vi "LED State Implem.vi"(1 "LED State":T1(ring)=enum."Balancing") -> ()   [LabVIEW 2020]
uses:
  <vilib>/Rock Robotics/WPI/DriverStation/WPI_DriverStationRobotMode2.ctl
  <vilib>/Rock Robotics/Network Tables/NT Read Boolean.vi
  <vilib>/Rock Robotics/Network Tables/NT Read Number.vi
  Robot Global Data.vi
panel:
  out "size(s)":i32
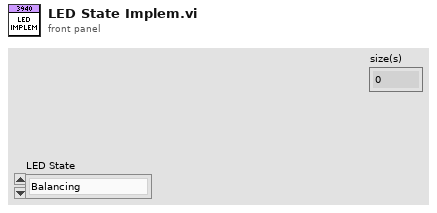
[diagram p1: front panel]
types:
  T1 = enum16{"Default", "Cone", "Cube", "Acquired", "Auto Red", "Auto Blue", "Balancing"}
  T2 = typedef "WPI_DriverStationRobotMode2.ctl" = enum16{"Autonomous Disabled", "Autonomous Enabled", "Teleop Disabled", "Teleop Enabled", "Disconnected", "Finish", "Test Disabled", "Test Enabled", "Emergency Stopped"}
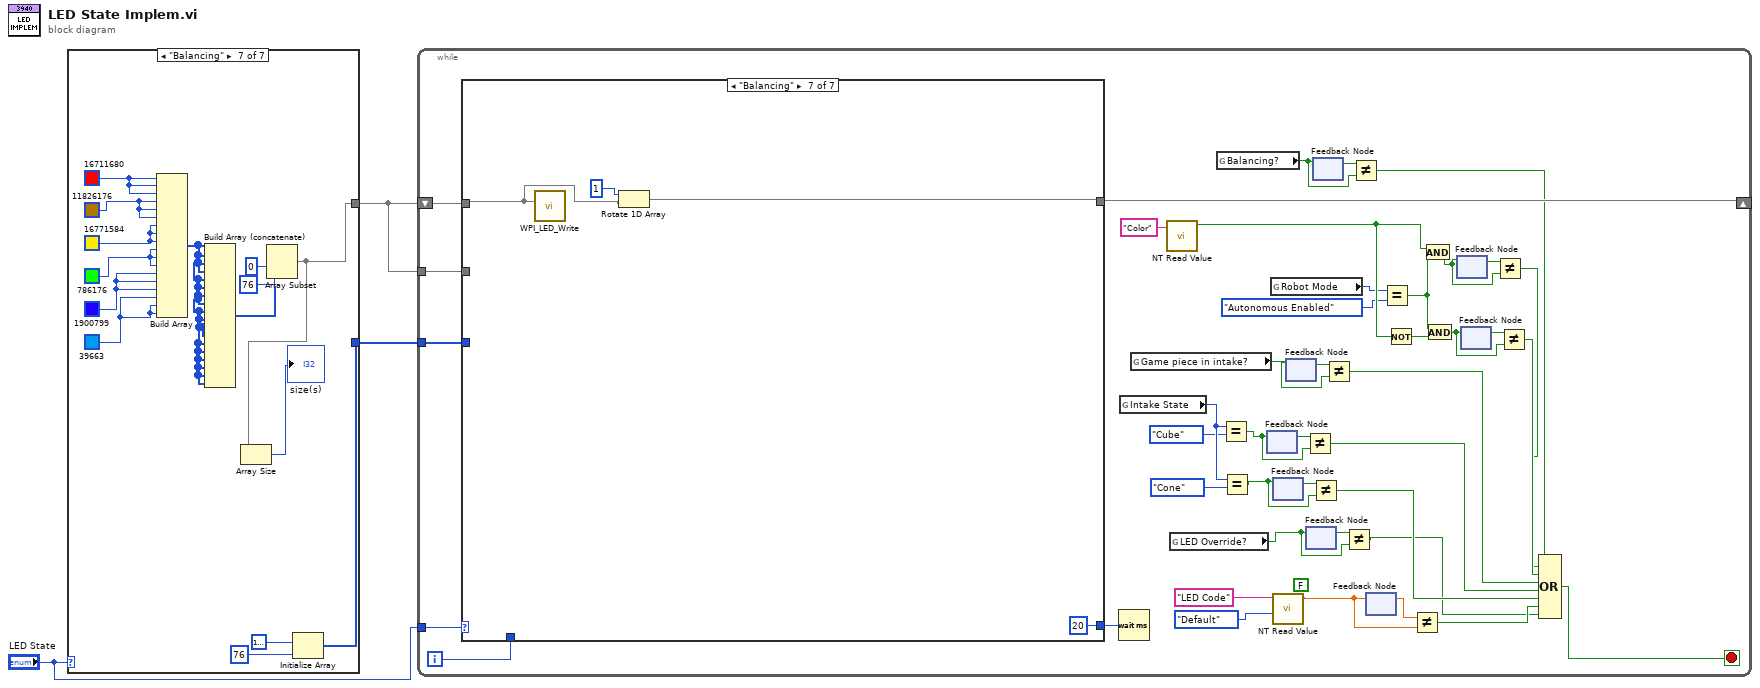
[diagram p0: block diagram]
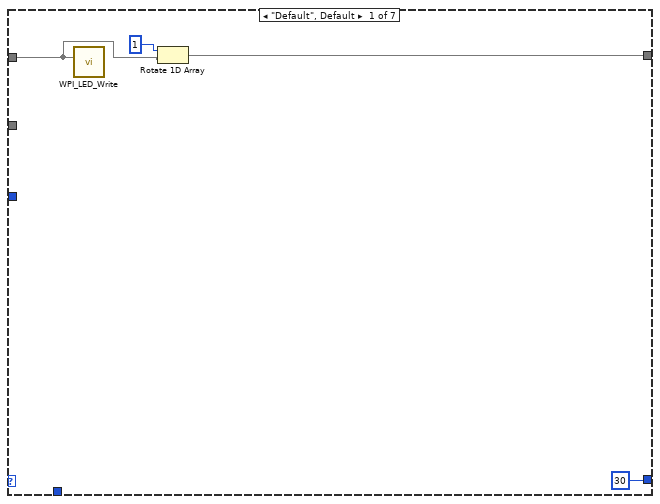
[diagram p2: hidden frame]
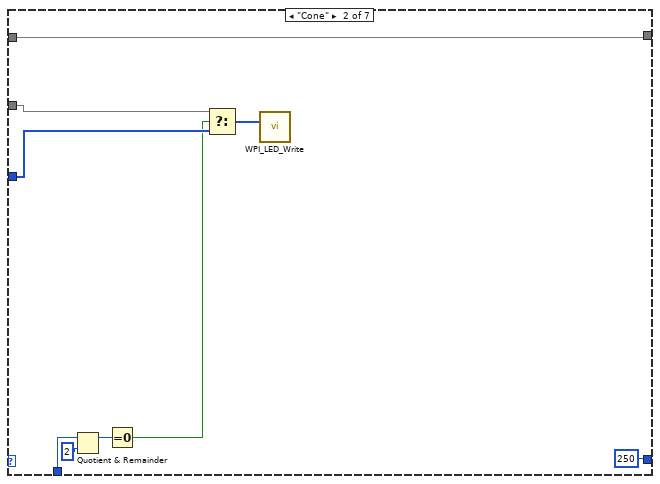
[diagram p3: hidden frame]
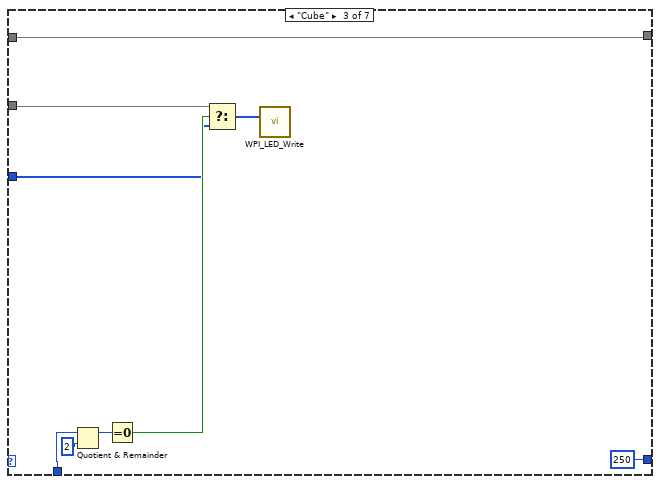
[diagram p4: hidden frame]
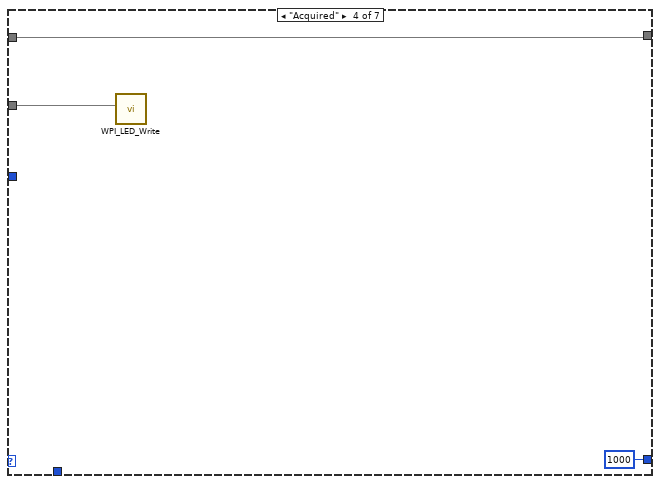
[diagram p5: hidden frame]
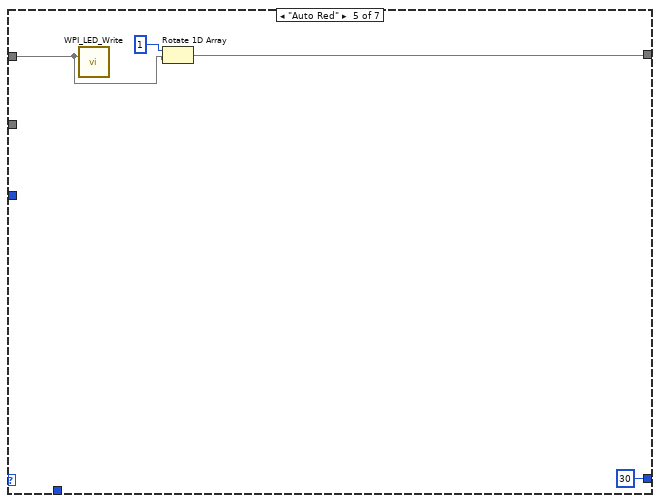
[diagram p6: hidden frame]
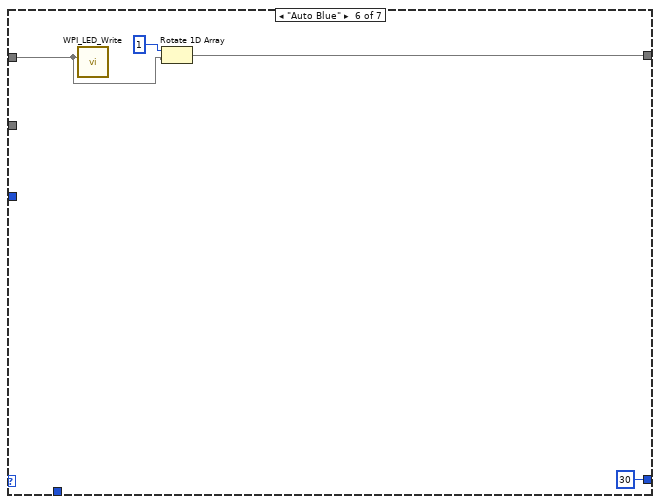
[diagram p7: hidden frame]
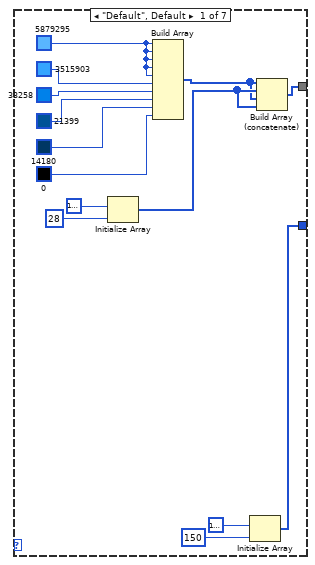
[diagram p8: hidden frame]
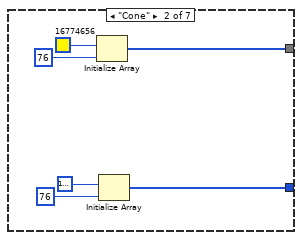
[diagram p9: hidden frame]
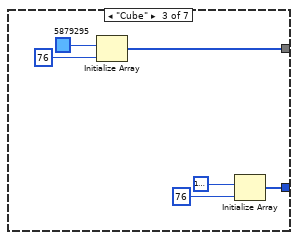
[diagram p10: hidden frame]
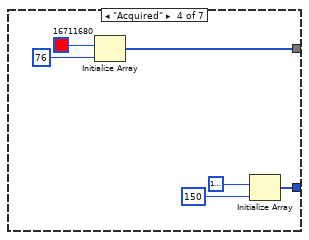
[diagram p11: hidden frame]
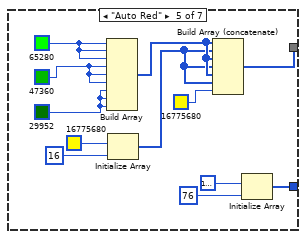
[diagram p12: hidden frame]
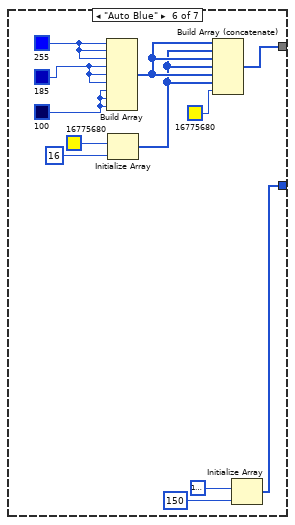
[diagram p13: hidden frame]
diagram:
  n1 = case shown="\"Balancing\"" "LED State" {
    tunnel: [w15 w21 w27 w33 w39 w51 w60] -> w2
    tunnel: [w12 w18 w24 w30 w45 w57 w72] -> w1
    frame "Default", Default {
      w11 = u32 5879295
      n2 = Initialize Array(u32 16777216, 28 ("dimension size")) -> (w5:u32[])
      n3 = Build Array(w11, w11, w11, w11, w11, u32 3515903, u32 33258, u32 21399, u32 14180, u32 0) -> (w4:u32[])
      n4 = Initialize Array(u32 16777216, 150 ("dimension size")) -> (w12:u32[])
      n5 = Build Array (concatenate)(w4, w5, w4, w5) -> (w15:u32[])
    }
    frame "Cone" {
      n6 = Initialize Array(u32 16774656, 76 ("dimension size")) -> (w21:u32[])
      n7 = Initialize Array(u32 16777216, 76 ("dimension size")) -> (w18:u32[])
    }
    frame "Cube" {
      n8 = Initialize Array(u32 5879295, 76 ("dimension size")) -> (w27:u32[])
      n9 = Initialize Array(u32 16777216, 76 ("dimension size")) -> (w24:u32[])
    }
    frame "Acquired" {
      n10 = Initialize Array(u32 16711680, 76 ("dimension size")) -> (w33:u32[])
      n11 = Initialize Array(u32 16777216, 150 ("dimension size")) -> (w30:u32[])
    }
    frame "Auto Red" {
      w42 = u32 29952
      w43 = u32 47360
      w44 = u32 65280
      n12 = Build Array(w44, w44, w44, w43, w43, w43, w42, w42, w42) -> (w38:u32[])
      n13 = Initialize Array(u32 16775680, 16 ("dimension size")) -> (w37:u32[])
      n14 = Build Array (concatenate)(w38, w37, w38, w37, w38, w37, u32 16775680) -> (w39:u32[])
      n15 = Initialize Array(u32 16777216, 76 ("dimension size")) -> (w45:u32[])
    }
    frame "Auto Blue" {
      w54 = u32 100
      w55 = u32 185
      w56 = u32 255
      n16 = Build Array(w56, w56, w56, w55, w55, w55, w54, w54, w54) -> (w50:u32[])
      n17 = Initialize Array(u32 16775680, 16 ("dimension size")) -> (w49:u32[])
      n18 = Build Array (concatenate)(w50, w49, w50, w49, w50, w49, u32 16775680) -> (w51:u32[])
      n19 = Initialize Array(u32 16777216, 150 ("dimension size")) -> (w57:u32[])
    }
    frame "Balancing" {
      w66 = u32 39663
      w67 = u32 1900799
      w68 = u32 786176
      w69 = u32 16771584
      w70 = u32 11826176
      w71 = u32 16711680
      n20 = Build Array(w71, w71, w71, w70, w70, w70, w69, w69, w69, w68, w68, w68, w67, w67, w67, w66, w66, w66) -> (w61:u32[])
      n21 = Build Array (concatenate)(w61, w61, w61, w61, w61, w61, w61, w61, w61, w61, w61, w61, w61, w61, w61, w61, w61, w61) -> (w62:u32[])
      n22 = Array Subset(array=w62, index=0, length=76) -> (w60:u32[])
      n23 = Array Size(array=w60) -> (size(s)=→"size(s)":i32)
      n24 = Initialize Array(u32 16777216, 76 ("dimension size")) -> (w72:u32[])
    }
  }
  n25 = while {
    tunnel: "LED State" -> [w117]
    shift-right: [w115] -> _
    shift-left: w2 -> [w116]
    tunnel: w2 -> [w114]
    tunnel: w1 -> [w111]
    i -> [w113]
    stop <- w101 stop-if-true
    (unwired) FALSE ("value")
    n26 = case shown="\"Balancing\"" w117 {
      tunnel: w116 -> [w121 w123 w139 w142 w144 w148 w152]
      tunnel: [w119 w123 w139 w142 w143 w147 w151] -> w115
      tunnel: w114 -> [_ w126 w134 w141 _ _ _]
      tunnel: w113 -> [_ w130 w132 _ _ _ _]
      tunnel: [30 250 250 1000 30 30 20] -> w112
      tunnel: w111 -> [_ w125 w135 _ _ _ _]
      frame "Default", Default {
        n27 = call <vilib>:"WPI_LED_Write.vi"("Color Array"=w121) -> ()  [unwired: 10 in, 1 out]
        n28 = Rotate 1D Array(1:w121, 2:1 ("n")) -> (0:w119:u32[])
      }
      frame "Cone" {
        n29 = Quotient & Remainder(x=w130, y=2) -> (x-y*floor(x/y)=w128:i32)  [unwired: 1 out]
        n30 = Equal To 0?(x=w128) -> (x = 0?=w124:bool)
        n31 = Select(t=w126, s=w124, f=w125) -> (s? t:f=w127:u32[])
        n32 = call <vilib>:"WPI_LED_Write.vi"("Color Array"=w127) -> ()  [unwired: 10 in, 1 out]
      }
      frame "Cube" {
        n33 = Quotient & Remainder(x=w132, y=2) -> (x-y*floor(x/y)=w137:i32)  [unwired: 1 out]
        n34 = Equal To 0?(x=w137) -> (x = 0?=w136:bool)
        n35 = Select(t=w134, s=w136, f=w135) -> (s? t:f=w133:u32[])
        n36 = call <vilib>:"WPI_LED_Write.vi"("Color Array"=w133) -> ()  [unwired: 10 in, 1 out]
      }
      frame "Acquired" {
        n37 = call <vilib>:"WPI_LED_Write.vi"("Color Array"=w141) -> ()  [unwired: 10 in, 1 out]
      }
      frame "Auto Red" {
        n38 = call <vilib>:"WPI_LED_Write.vi"("Color Array"=w144) -> ()  [unwired: 10 in, 1 out]
        n39 = Rotate 1D Array(1:w144, 2:1 ("n")) -> (0:w143:u32[])
      }
      frame "Auto Blue" {
        n40 = call <vilib>:"WPI_LED_Write.vi"("Color Array"=w148) -> ()  [unwired: 10 in, 1 out]
        n41 = Rotate 1D Array(1:w148, 2:1 ("n")) -> (0:w147:u32[])
      }
      frame "Balancing" {
        n42 = call <vilib>:"WPI_LED_Write.vi"("Color Array"=w152) -> ()  [unwired: 10 in, 1 out]
        n43 = Rotate 1D Array(1:w152, 2:1 ("n")) -> (0:w151:u32[])
      }
    }
    n44 = Wait (ms)(milliseconds to wait=w112) -> ()  [unwired: 1 out]
    n45 = global read "Robot Global Data.vi" "Intake State"() -> (w104:enum16{"Cone", "Cube", "Cube Handoff", "Stow"})
    n46 = global read "Robot Global Data.vi" "Game piece in intake?"() -> (w89:bool)
    n47 = call-poly <vilib>:"NT Read Value.vi"("name"="Color") -> ("value"=w110:bool)  [unwired: 8 in, 2 out]
    n48 = global read "Robot Global Data.vi" "LED Override?"() -> (w76:bool)
    n49 = global read "Robot Global Data.vi" "Balancing?"() -> (w80:bool)
    n50 = Equal?(x=w104, y=enum16{"Cone", "Cube", "Cube Handoff", "Stow"}."Cube" ("Intake State")) -> (x = y?=w92:bool)
    n51 = Equal?(x=w104, y=enum16{"Cone", "Cube", "Cube Handoff", "Stow"}."Cone" ("Intake State")) -> (x = y?=w95:bool)
    n52 = feedback #1() -> (w93:bool)  [unwired: 1 in]
    n53 = feedback-in #1(w92) -> ()
    n54 = global read "Robot Global Data.vi" "Robot Mode"() -> (w107:T2)
    n55 = feedback #2() -> (w96:bool)  [unwired: 1 in]
    n56 = feedback-in #2(w95) -> ()
    n57 = call-poly <vilib>:"NT Read Value.vi"("default value"=T1."Default" ("t"), "name"="LED Code") -> ("value"=w97:dbl)  [unwired: 7 in, 2 out]
    n58 = feedback #3() -> (w90:bool)  [unwired: 1 in]
    n59 = feedback-in #3(w89) -> ()
    n60 = Not Equal?(x=w93, y=w92) -> (x != y?=w91:bool)
    n61 = feedback #4() -> (w77:bool)  [unwired: 1 in]
    n62 = feedback-in #4(w76) -> ()
    n63 = Not Equal?(x=w96, y=w95) -> (x != y?=w94:bool)
    n64 = feedback #5() -> (w81:bool)  [unwired: 1 in]
    n65 = feedback-in #5(w80) -> ()
    n66 = Not Equal?(x=w90, y=w89) -> (x != y?=w88:bool)
    n67 = Not Equal?(x=w77, y=w76) -> (x != y?=w75:bool)
    n68 = Not Equal?(x=w81, y=w80) -> (x != y?=w79:bool)
    n69 = feedback-in #6(w97) -> ()
    n70 = feedback #6() -> (w98:dbl)  [unwired: 1 in]
    n71 = Equal?(x=w107, y=WPI_DriverStationRobotMode2."Autonomous Enabled" ("Robot Mode")) -> (x = y?=w108:bool)
    n72 = Not(x=w110) -> (.not. x?=w109:bool)
    n73 = Not Equal?(x=w98, y=w97) -> (x != y?=w78:bool)
    n74 = And(x=w110, y=w108) -> (x .and. y?=w83:bool)
    n75 = And(x=w108, y=w109) -> (x .and. y?=w86:bool)
    n76 = feedback #7() -> (w84:bool)  [unwired: 1 in]
    n77 = feedback-in #7(w83) -> ()
    n78 = feedback #8() -> (w87:bool)  [unwired: 1 in]
    n79 = feedback-in #8(w86) -> ()
    n80 = Not Equal?(x=w84, y=w83) -> (x != y?=w82:bool)
    n81 = Not Equal?(x=w87, y=w86) -> (x != y?=w85:bool)
    n82 = Compound Arithmetic op=OR(w79, w82, w85, w88, w91, w94, w78, w75) -> (w101:bool)
  }
